vi "运维调试_河水净化.vi"() -> ()   [LabVIEW 2016, in "PLC.lvlib"]
uses:
  PLC.lvlib
  control/switch.ctl
  <vilib>/Utility/miscctls.llb/LVPointTypeDef.ctl
panel:
  out "R133":i16 caption="絮凝剂润洗时间"
  in  "返回":T1
  out "R132":i16 caption="精密过滤清洗时间"
  out "R131":i16 caption="前置过滤清洗时间"
  out "R130":i16 caption="搅拌桶搅拌时间"
  out "R129":i16 caption="搅拌桶进样超时时间"
  out "R128":i16 caption="搅拌桶润洗时间"
  out "R127":i16 caption="絮凝剂进样时间"
  out "R126":i16 caption="搅拌桶排液时间"
  in  "河水净化启用":bool
  in  "参数设置":T1
  in  "停止":T1
  in  "过滤清洗":T1
  in  "过滤":T1
  in  "润洗进样":T1
  out "X12":bool caption="搅拌桶高液位"
  out "X11":bool caption="搅拌桶低液位"
  out "R29":u16
  out "R28":u16
  out "R14":u16
  out "R13":u16
  in  "Y1":T1
  in  "Y0":T1
  in  "Y16":T1
  in  "Y15":T1
  out "R77":u16
  in  "Y39":T1
  out "R76":u16
  in  "Y38":T1
  out "R75":u16
  in  "Y37":T1
  out "R74":u16
  in  "Y36":T1
  out "R73":u16
  in  "Y35":T1
  out "R72":u16
  in  "Y34":T1
  out "R71":u16
  in  "Y33":T1
  out "多列列表框":i32(listbox)
  out "R70":u16
  in  "Y32":T1
  # "S"
  # "S"
  # "S"
  # "S"
  # "S"
  # "S"
  # "S"
  # "S"
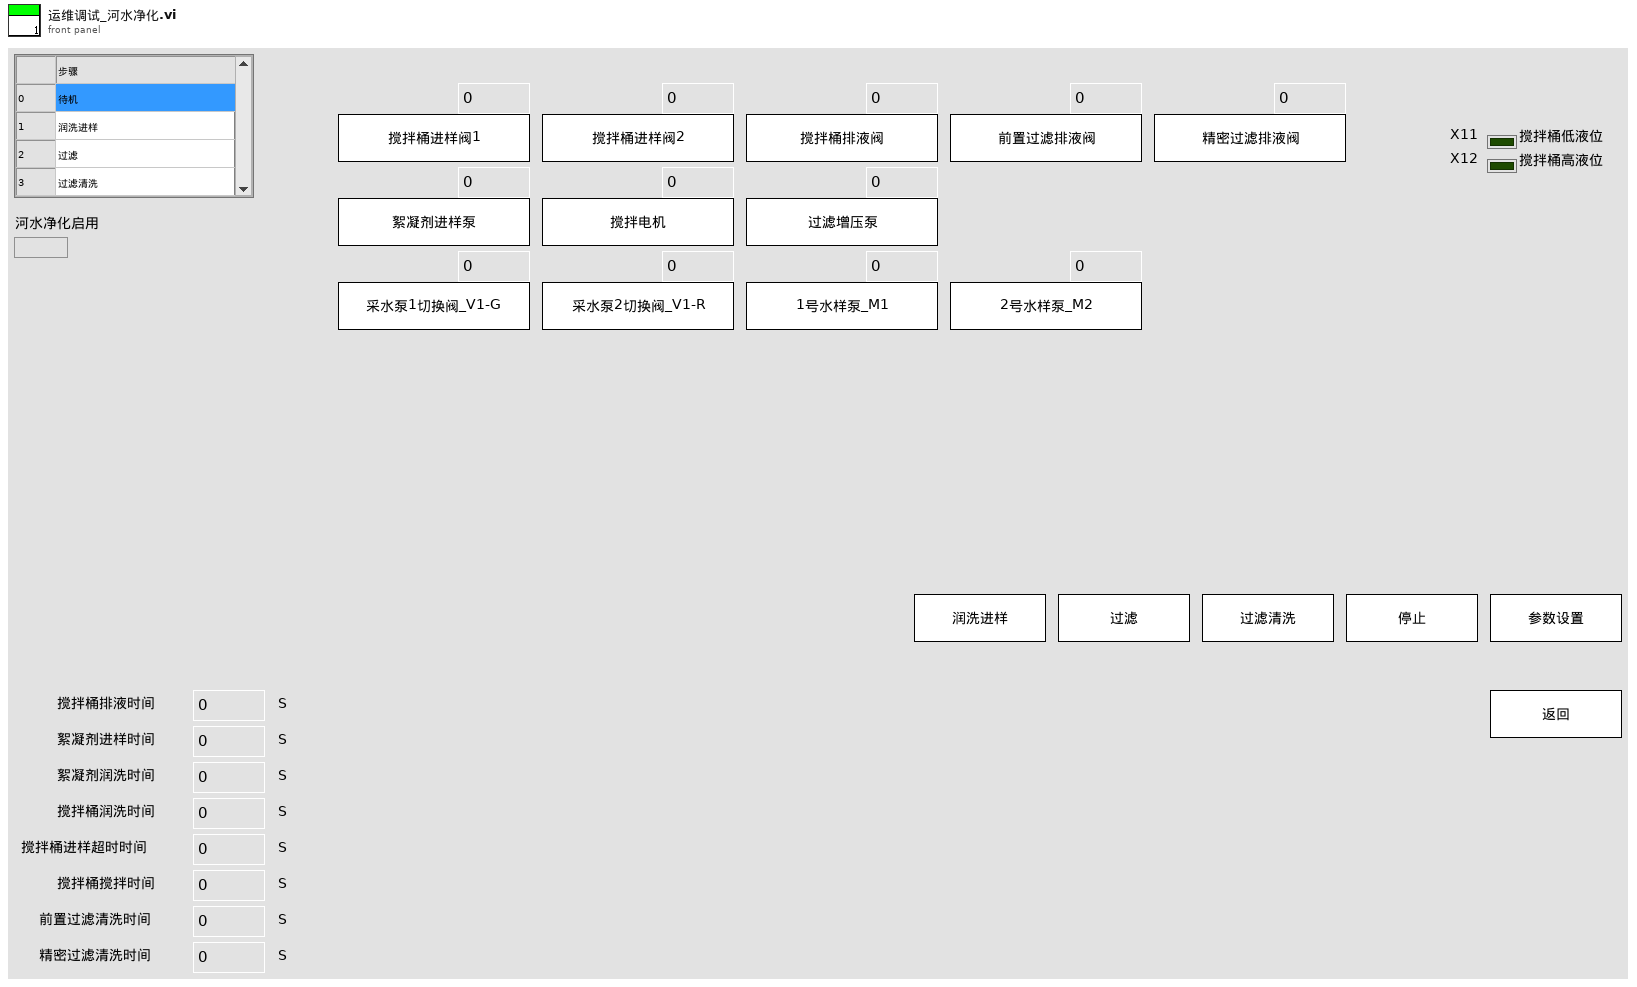
[diagram p1: front panel]
types:
  T1 = typedef "PLC.lvlib/switch.ctl" = bool
  T2 = typedef "LVPointTypeDef.ctl" = cluster{"Horizontal":i16, "Vertical":i16}
  T3 = cluster{"R100":i16, "R101":i16, "R102":i16, "R103":i16, "R104":i16, "R105":i16, "R106":i16, "R107":i16, "R108":i16, "R109":i16, "R110":i16, "R111":i16, "R112":i16, "R113":i16, "R114":i16, "R115":i16, "R116":i16, "R117":i16, "R118":i16, "R119":i16, "R120":i16, "R121":i16, "R122":i16, "R123":i16, "R124":i16, "R125":i16, "R126":i16, "R127":i16, "R128":i16, "R129":i16, "R130":i16, "R131":i16, "R132":i16, "R133":i16}
  T4 = cluster{"R0":i16, "R1":i16, "R2":i16, "R3":i16, "R4":i16, "R5":i16, "R6":i16, "R7":i16, "R8":i16, "R9":i16, "R10":i16, "R11":i16, "R12":i16, "R13":i16, "R14":i16, "R15":i16, "R16":i16, "R17":i16, "R18":i16, "R19":i16, "R20":i16, "R21":i16, "R22":i16, "R23":i16, "R24":i16, "R25":i16, "R26":i16, "R27":i16, "R28":i16, "R29":i16, "R30":i16, "R31":i16, "R32":i16, "R33":i16, "R34":i16, "R35":i16, "R36":i16, "R37":i16, "R38":i16, "R39":i16, "R40":i16, "R41":i16, "R42":i16, "R43":i16, "R44":i16, "R45":i16, "R46":i16, "R47":i16, "R48":i16, "R49":i16, "R50":i16, "R51":i16, "R52":i16, "R53":i16, "R54":i16, "R55":i16, "R56":i16, "R57":i16, "R58":i16, "R59":i16, "R60":i16, "R61":i16, "R62":i16, "R63":i16, "R64":i16, "R65":i16, "R66":i16, "R67":i16, "R68":i16, "R69":i16, "R70":i16, "R71":i16, "R72":i16, "R73":i16, "R74":i16, "R75":i16, "R76":i16, "R77":i16, "R78":i16, "R79":i16}
  T5 = cluster{"命令":string, "数据":cluster{"starting address":u16, "holding register values":u16[]}}
  T6 = cluster{"命令":string, "data":cluster{"starting address":u16, "coil values":bool[]}}
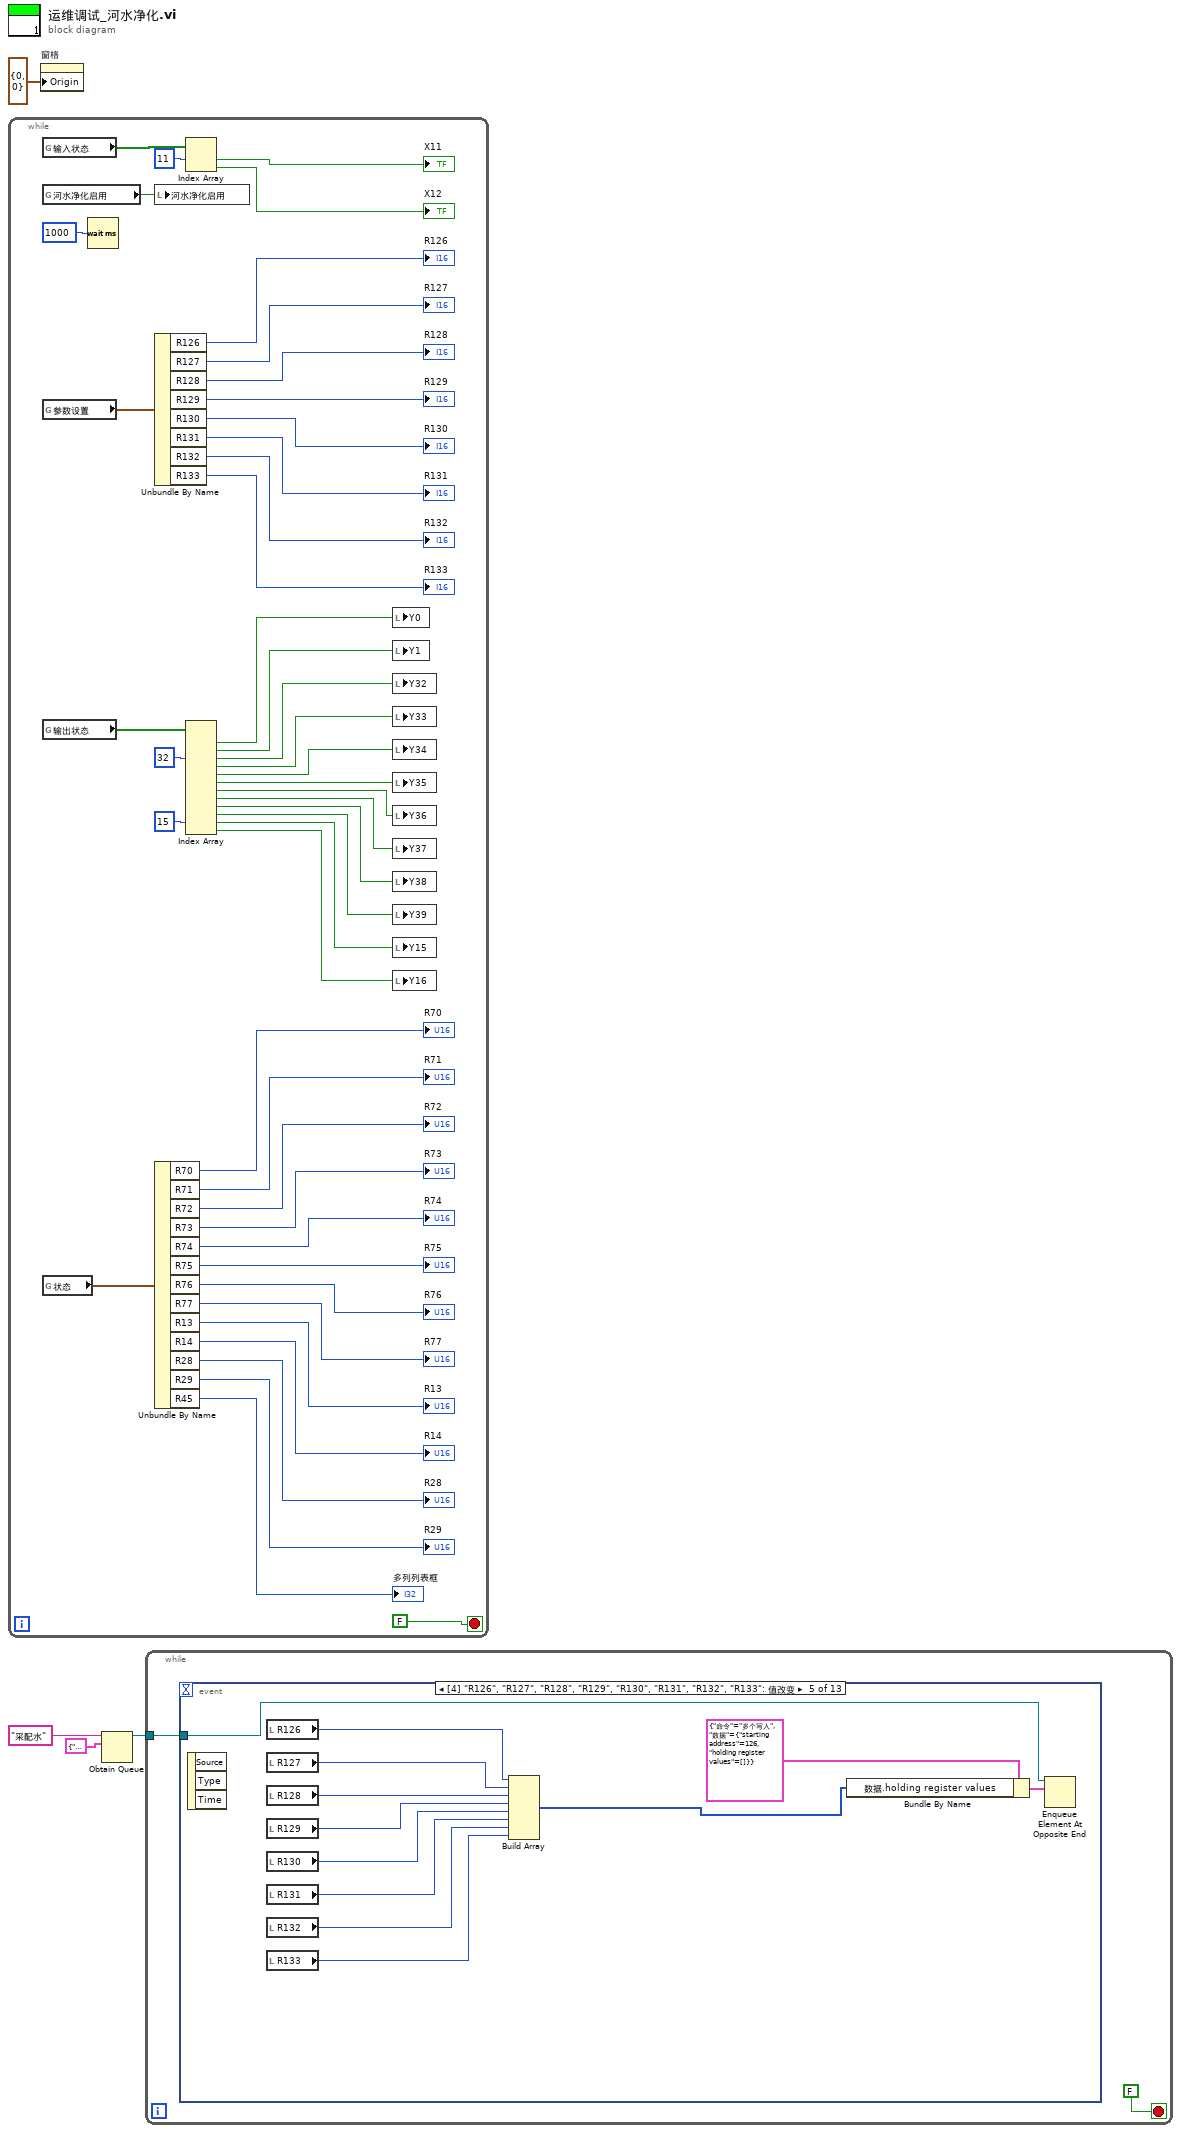
[diagram p0: block diagram]
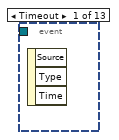
[diagram p2: hidden frame]
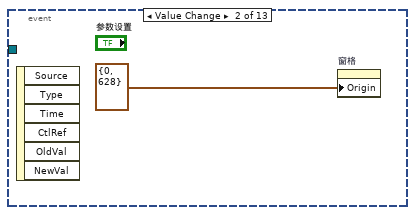
[diagram p3: hidden frame]
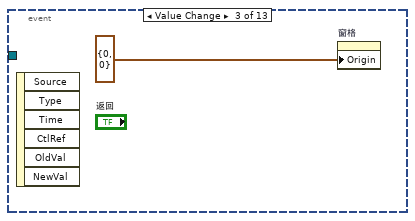
[diagram p4: hidden frame]
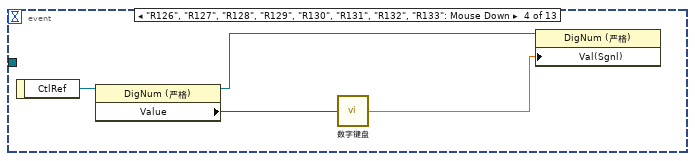
[diagram p5: hidden frame]
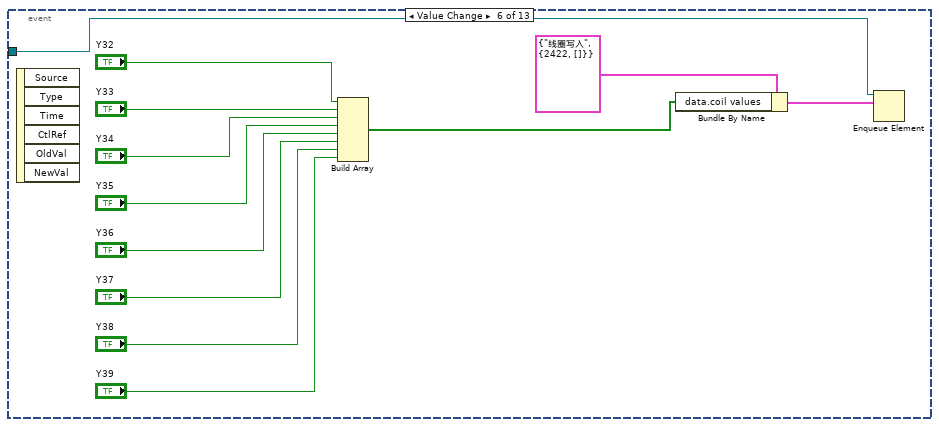
[diagram p6: hidden frame]
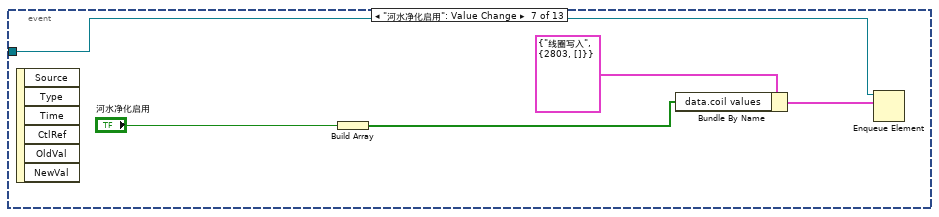
[diagram p7: hidden frame]
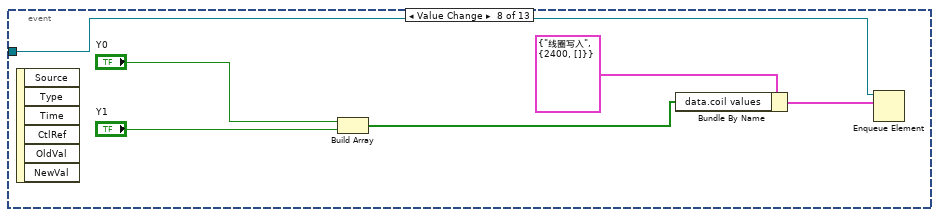
[diagram p8: hidden frame]
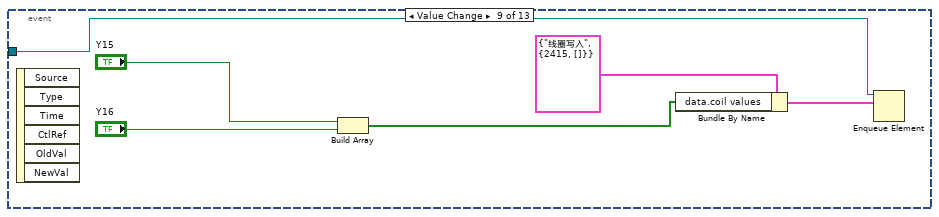
[diagram p9: hidden frame]
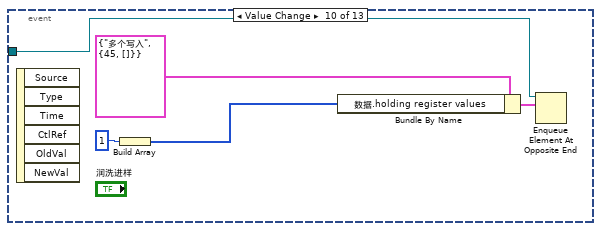
[diagram p10: hidden frame]
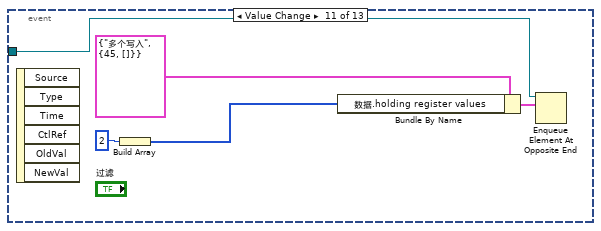
[diagram p11: hidden frame]
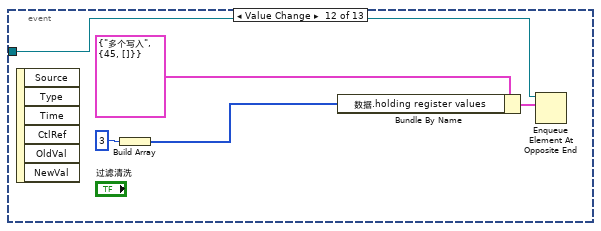
[diagram p12: hidden frame]
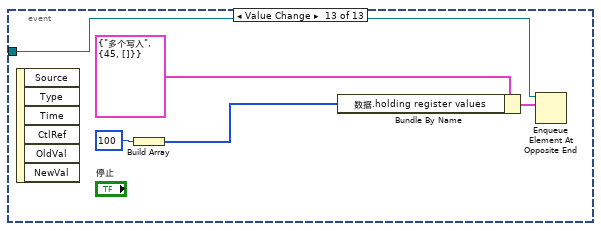
[diagram p13: hidden frame]
diagram:
  n1 = while {
    stop <- FALSE stop-if-true
    n2 = global read "采配水全局变量.vi" "输入状态"() -> (w47:bool[])
    n3 = global read "采配水全局变量.vi" "河水净化启用"() -> (w15:bool)
    n4 = global read "采配水全局变量.vi" "参数设置"() -> (w14:T3)
    n5 = global read "采配水全局变量.vi" "输出状态"() -> (w42:bool[])
    n6 = global read "采配水全局变量.vi" "状态"() -> (w33:T4)
    n7 = Wait (ms)(milliseconds to wait=u32 1000 ("等待时间（毫秒）")) -> ()  [unwired: 1 out]
    n8 = local write "河水净化启用"(w15) -> ()
    n9 = Unbundle By Name(w14) -> ("R126"=→"R126":i16, "R127"=→"R127":i16, "R128"=→"R128":i16, "R129"=→"R129":i16, "R130"=→"R130":i16, "R131"=→"R131":i16, "R132"=→"R132":i16, "R133"=→"R133":i16)
    n10 = Unbundle By Name(w33) -> ("R70"=→"R70":i16, "R71"=→"R71":i16, "R72"=→"R72":i16, "R73"=→"R73":i16, "R74"=→"R74":i16, "R75"=→"R75":i16, "R76"=→"R76":i16, "R77"=→"R77":i16, "R13"=→"R13":i16, "R14"=→"R14":i16, "R28"=→"R28":i16, "R29"=→"R29":i16, "R45"=→"多列列表框":i16)
    n11 = Index Array(array=w47, index #1=11 ("索引")) -> (element #1=→"X11":bool, element #2=→"X12":bool)  [unwired: 1 in]
    n12 = Index Array(array=w42, index #3=32 ("索引"), index #11=15 ("索引")) -> (element #1=w20:bool, element #2=w19:bool, element #3=w41:bool, element #4=w40:bool, element #5=w39:bool, element #6=w38:bool, element #7=w37:bool, element #8=w36:bool, element #9=w35:bool, element #10=w34:bool, element #11=w17:bool, element #12=w16:bool)  [unwired: 10 in]
    n13 = local write "Y0"(w20) -> ()
    n14 = local write "Y1"(w19) -> ()
    n15 = local write "Y32"(w41) -> ()
    n16 = local write "Y33"(w40) -> ()
    n17 = local write "Y34"(w39) -> ()
    n18 = local write "Y35"(w38) -> ()
    n19 = local write "Y36"(w37) -> ()
    n20 = local write "Y37"(w36) -> ()
    n21 = local write "Y38"(w35) -> ()
    n22 = local write "Y39"(w34) -> ()
    n23 = local write "Y15"(w17) -> ()
    n24 = local write "Y16"(w16) -> ()
  }
  n25 = property on="窗格" class="Pane"("Origin"=T2 {"Horizontal"=0, "Vertical"=0} ("原点")) -> ()  [unwired: 2 in, 2 out]
  n26 = Obtain Queue(name (unnamed)="采配水" ("名称（未命名）"), element data type=cluster{"命令":string, "数据":variant} {"命令"="", "数据"=variant}) -> (queue out=w1:refnum<queue>)  [unwired: 3 in, 2 out]
  n27 = while {
    tunnel: w1 -> [w51]
    stop <- FALSE stop-if-true
    n28 = event shown="[4] \"R126\", \"R127\", \"R128\", \"R129\", \"R130\", \"R131\", \"R132\", \"R133\": 值改变" {
      selector: _ -> [_ _ _ _ _ _ _ _ _ _ _ _ _]
      dyn-events: _ -> [_ _ _ _ _ _ _ _ _ _ _ _ _]
      timeout: _ -> [_ _ _ _ _ _ _ _ _ _ _ _ _]
      tunnel: w51 -> [_ _ _ _ w67 w79 w84 w90 w96 w101 w106 w111 w116]
      event Timeout {
        n29 = event-data() -> ()  [unwired: 1 in, 3 out]
      }
      event Value Change {
        n30 = event-data() -> ()  [unwired: 1 in, 6 out]
        n31 = property on="窗格" class="Pane"("Origin"=T2 {"Horizontal"=0, "Vertical"=628} ("原点")) -> ()  [unwired: 2 in, 2 out]
      }
      event Value Change {
        n32 = event-data() -> ()  [unwired: 1 in, 6 out]
        n33 = property on="窗格" class="Pane"("Origin"=T2 {"Horizontal"=0, "Vertical"=0} ("原点")) -> ()  [unwired: 2 in, 2 out]
      }
      event "R126", "R127", "R128", "R129", "R130", "R131", "R132", "R133": Mouse Down {
        n34 = event-data() -> ("CtlRef"=w57:refnum<vi>)  [unwired: 1 in]
        n35 = property class="DigNum (严格)"(reference=w57) -> (reference out=w56:refnum<vi>, "Value"=w55:i16)  [unwired: 1 in, 1 out]
        n36 = call "数字键盘.vi"("OldNumber"=w55) -> ("NewNumber"=w54:sgl)
        n37 = property class="DigNum (严格)"(reference=w56, "Val(Sgnl)"=w54) -> ()  [unwired: 1 in, 2 out]
      }
      event "R126", "R127", "R128", "R129", "R130", "R131", "R132", "R133": Value Change {
        n38 = event-data() -> ()  [unwired: 1 in, 3 out]
        n39 = local read "R126"() -> (w66:i16)
        n40 = local read "R127"() -> (w64:i16)
        n41 = local read "R128"() -> (w63:i16)
        n42 = local read "R129"() -> (w62:i16)
        n43 = local read "R130"() -> (w61:i16)
        n44 = local read "R131"() -> (w60:i16)
        n45 = local read "R132"() -> (w59:i16)
        n46 = local read "R133"() -> (w58:i16)
        n47 = Build Array(w66, w64, w63, w62, w61, w60, w59, w58) -> (w65:i16[])
        n48 = Bundle By Name(cluster=T5 {"命令"="多个写入", "数据"={"starting address"=126, "holding register values"=[]}} ("元素"), "数据.holding register values"=w65) -> (w68:T5)
        n49 = Enqueue Element At Opposite End(queue=w67, element=w68) -> ()  [unwired: 2 in, 3 out]
      }
      event Value Change {
        n50 = event-data() -> ()  [unwired: 1 in, 6 out]
        n51 = Build Array("Y32", "Y33", "Y34", "Y35", "Y36", "Y37", "Y38", "Y39") -> (w78:T1[])
        n52 = Bundle By Name(cluster=T6 {"命令"="线圈写入", "data"={"starting address"=2422, "coil values"=[]}} ("元素"), "data.coil values"=w78) -> (w80:T6)
        n53 = Enqueue Element(queue=w79, element=w80) -> ()  [unwired: 2 in, 3 out]
      }
      event "河水净化启用": Value Change {
        n54 = event-data() -> ()  [unwired: 1 in, 6 out]
        n55 = Build Array("河水净化启用") -> (w82:bool[])
        n56 = Bundle By Name(cluster=T6 {"命令"="线圈写入", "data"={"starting address"=2803, "coil values"=[]}} ("元素"), "data.coil values"=w82) -> (w85:T6)
        n57 = Enqueue Element(queue=w84, element=w85) -> ()  [unwired: 2 in, 3 out]
      }
      event Value Change {
        n58 = event-data() -> ()  [unwired: 1 in, 6 out]
        n59 = Build Array("Y0", "Y1") -> (w89:T1[])
        n60 = Bundle By Name(cluster=T6 {"命令"="线圈写入", "data"={"starting address"=2400, "coil values"=[]}} ("元素"), "data.coil values"=w89) -> (w91:T6)
        n61 = Enqueue Element(queue=w90, element=w91) -> ()  [unwired: 2 in, 3 out]
      }
      event Value Change {
        n62 = event-data() -> ()  [unwired: 1 in, 6 out]
        n63 = Build Array("Y15", "Y16") -> (w95:T1[])
        n64 = Bundle By Name(cluster=T6 {"命令"="线圈写入", "data"={"starting address"=2415, "coil values"=[]}} ("元素"), "data.coil values"=w95) -> (w97:T6)
        n65 = Enqueue Element(queue=w96, element=w97) -> ()  [unwired: 2 in, 3 out]
      }
      event Value Change {
        n66 = event-data() -> ()  [unwired: 1 in, 6 out]
        n67 = Build Array(1) -> (w100:i32[])
        n68 = Bundle By Name(cluster=T5 {"命令"="多个写入", "数据"={"starting address"=45, "holding register values"=[]}} ("元素"), "数据.holding register values"=w100) -> (w102:T5)
        n69 = Enqueue Element At Opposite End(queue=w101, element=w102) -> ()  [unwired: 2 in, 3 out]
      }
      event Value Change {
        n70 = event-data() -> ()  [unwired: 1 in, 6 out]
        n71 = Build Array(2) -> (w105:i32[])
        n72 = Bundle By Name(cluster=T5 {"命令"="多个写入", "数据"={"starting address"=45, "holding register values"=[]}} ("元素"), "数据.holding register values"=w105) -> (w107:T5)
        n73 = Enqueue Element At Opposite End(queue=w106, element=w107) -> ()  [unwired: 2 in, 3 out]
      }
      event Value Change {
        n74 = event-data() -> ()  [unwired: 1 in, 6 out]
        n75 = Build Array(3) -> (w110:i32[])
        n76 = Bundle By Name(cluster=T5 {"命令"="多个写入", "数据"={"starting address"=45, "holding register values"=[]}} ("元素"), "数据.holding register values"=w110) -> (w112:T5)
        n77 = Enqueue Element At Opposite End(queue=w111, element=w112) -> ()  [unwired: 2 in, 3 out]
      }
      event Value Change {
        n78 = event-data() -> ()  [unwired: 1 in, 6 out]
        n79 = Build Array(100) -> (w115:i32[])
        n80 = Bundle By Name(cluster=T5 {"命令"="多个写入", "数据"={"starting address"=45, "holding register values"=[]}} ("元素"), "数据.holding register values"=w115) -> (w117:T5)
        n81 = Enqueue Element At Opposite End(queue=w116, element=w117) -> ()  [unwired: 2 in, 3 out]
      }
    }
  }
